vi "conversion_init.vi"() -> (0 "Signal list":refnum<k21>[](array[refnum]), 1 "CAN2 conversion session":T1, 2 "CAN1 conversion session":T1)   [LabVIEW 2017]
uses:
  <vilib>/xnet/xnet.llb/XNET Create Session (Conversion).vi
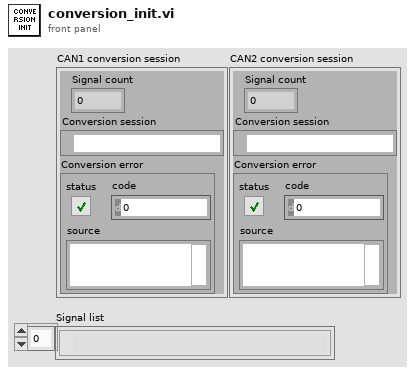
[diagram p1: front panel]
types:
  T1 = cluster{"Signal count":i32, "Conversion session":refnum<k21>, "Conversion error":errorcluster}
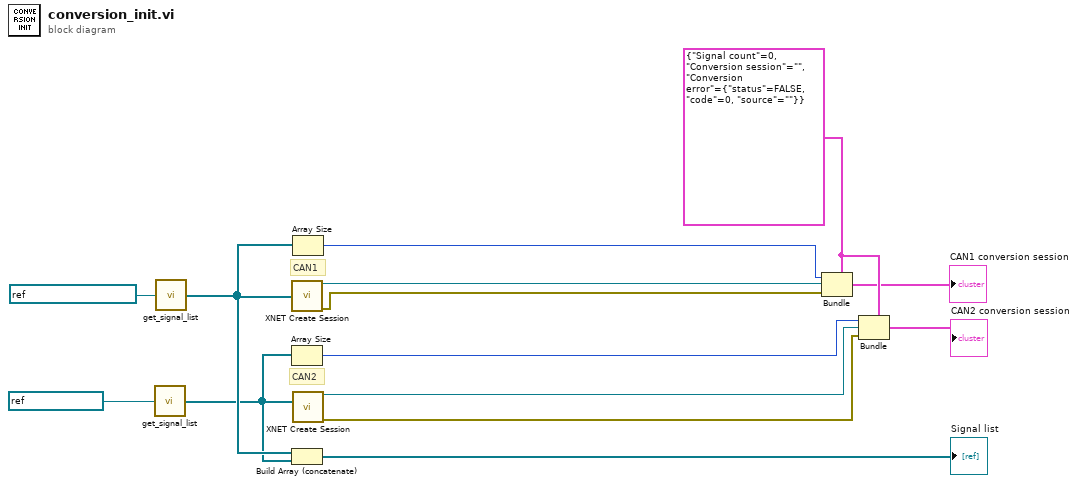
[diagram p0: block diagram]
diagram:
  w6 = T1 {"Signal count"=0, "Conversion session"="", "Conversion error"={"status"=FALSE, "code"=0, "source"=""}}
  # "CAN2"
  # "CAN1"
  n1 = call "get_signal_list.vi"("Refnum in"=refnum<k21> "BRUTUS_dbc") -> ("Sigs"=w10:refnum<k21>[])
  n2 = call "get_signal_list.vi"("Refnum in"=refnum<k21> "CAN1_matrix_2022" ("XNET Database")) -> ("Sigs"=w12:refnum<k21>[])
  n3 = call-poly <vilib>:"XNET Create Session.vi"("signal list"=w12) -> ("session out"=w8:refnum<k21>, "error out"=w7:errorcluster)  [unwired: 13 in]
  n4 = Array Size(array=w10) -> (size(s)=w5:i32)
  n5 = Build Array (concatenate)(w12, w10) -> (→"Signal list":refnum<k21>[])
  n6 = Array Size(array=w12) -> (size(s)=w9:i32)
  n7 = call-poly <vilib>:"XNET Create Session.vi"("signal list"=w10) -> ("session out"=w4:refnum<k21>, "error out"=w3:errorcluster)  [unwired: 13 in]
  n8 = Bundle(cluster=w6, "Signal count"=w9, "Conversion session"=w8, "Conversion error"=w7) -> (→"CAN1 conversion session":T1)
  n9 = Bundle(cluster=w6, "Signal count"=w5, "Conversion session"=w4, "Conversion error"=w3) -> (→"CAN2 conversion session":T1)
